vi "Minify jsonrpc id.vi"(8 "error in (no error)":errorcluster, 11 "<JSON> Requests":string) -> (0 "error out":errorcluster, 3 "<JSON>":string)   [LabVIEW 2019, in "Instrument.lvclass"]
uses:
  Instrument.lvclass
  <vilib>/JDP Science/JSONtext/JSONtext.lvlib
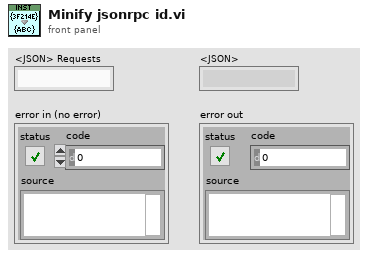
[diagram p1: front panel]
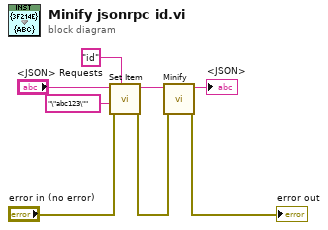
[diagram p0: block diagram]
diagram:
  n1 = call <vilib>:"Set Item.vi"("$Path or Item Name"="id", "error in (no error)"="error in (no error)", "JSON to Insert"="\"abc123\"", "JSON"="<JSON> Requests") -> ("error out"=w7:errorcluster, "<JSON>"=w5:string)  [unwired: 4 in, 1 out]
  n2 = call <vilib>:"Minify.vi"("error in (no error)"=w7, "JSON"=w5) -> ("error out"=→"error out":errorcluster, "<JSON>"=→"<JSON>":string)  [unwired: 7 in, 1 out]
